vi "Format S Parameters For Display.vi"(0 "S Parameters":cdb[](array[numeric])) -> (4 "S Parameters For Display":dbl[](array[numeric]))   [LabVIEW 2023, in "RFFixtureCharact.Public.lvlib" / "Vector Abstract Path.lvclass"]
uses:
  Vector Abstract Path.lvclass
  Vector Abstract Path.lvclass/Vector Abstract Path.ctl
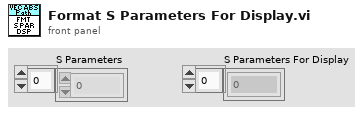
[diagram p1: front panel]
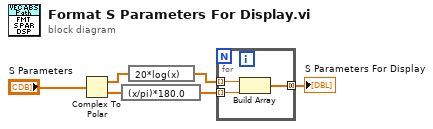
[diagram p0: block diagram]
diagram:
  n1 = Complex To Polar(r * e^(i*theta)="S Parameters") -> (r=w6:dbl[], theta=w4:dbl[])
  n2 = expression code="(x/pi)*180.0" ("radians to degrees")(w4) -> (w3:dbl[])
  n3 = expression code="20*log(x)"(w6) -> (w5:dbl[])
  n4 = for {
    tunnel: w5 -> [w9] mode=indexing
    tunnel: w3 -> [w8] mode=indexing
    tunnel: [w7] -> w1 mode=concatenating
    n5 = Build Array(w9, w8) -> (w7:dbl[])
  }
  "S Parameters For Display" <- w1
